vi "PH_Beckhoff_StepMot.ProcCases.vi"(0 "i ref in":refnum<vi>, 1 "selector":string, 2 "Data":T1, 3 "call cluster":T2={"Object"="", "Selector"="", "CallType"=enum."synchronous", "Async Object"="", "Async Selector"="", "Data Descriptor"="", "Data"=[], "Error #"=0, "Expire"=0}, 5 "error in (no error)":errorcluster) -> (14 "i ref out":refnum<vi>, 17 "answer cluster":T2={"Object"="", "Selector"="", "CallType"=enum."synchronous", "Async Object"="", "Async Selector"="", "Data Descriptor"="", "Data"=[], "Error #"=0, "Expire"=0}, 19 "error out":errorcluster)   [LabVIEW 2014, in "PH_Beckhoff_StepMot.lvlib"]
doc: "This method is called by a process from within the default case in the event loop. The methods of a class that are linked to events will be called from THIS method. Add your code here."
uses:
  PH_Beckhoff_StepMot.lvlib
  CS_Core/CSSystem/CoreDefs/CoreDefs.call_type.ctl
  CS_Core/BaseProcess/BaseProcess.descriptor string definition.ctl
  CS_Core/CSSystem/CoreDefs/CoreDefs.rawDataType.ctl
  PH_Beckhoff_StepMot.Axis Cluster.ctl
  instr.lib/Beckhoff/Specials/Step Motor Klemmen/Beckhoff.Step Motor - Motor Configuration.ctl
  instr.lib/Beckhoff/Read and Write Register/Step Motor Klemmen/Beckhoff.Step Motor - Feature Register 1.ctl
  instr.lib/Beckhoff/Read and Write Register/Step Motor Klemmen/Beckhoff.Step Motor - Feature Register 2.ctl
  PH_Basics/PH_PSDBWriter/PH_PSDBWriter.Thread Commands.ctl
  CS_Core/CSSystem/CoreLib/CoreLib.byte array 2 int.vi
  CS_Core/CSSystem/CoreLib/CoreLib.byte array 2 double.vi
  CS_Core/CSSystem/CoreLib/CoreLib.string 2 byte array.vi
  PH_Beckhoff/PH_Beckhoff.lvlib
  CS_Core/CSSystem/CoreLib/CoreLib.lvlib
  CS_Core/BaseProcess/BaseProcess.lvlib
  instr.lib/Beckhoff/Beckhoff - Driver np.lvlib
  PH_Basics/PH_Stepmotor_BaseClass/PH_Stepmotor_BaseClass.lvlib
  PH_Basics/PH_PSDBWriter/PH_PSDBWriter.lvlib
  CS_Core/CAEObj/CAEObj.lvlib
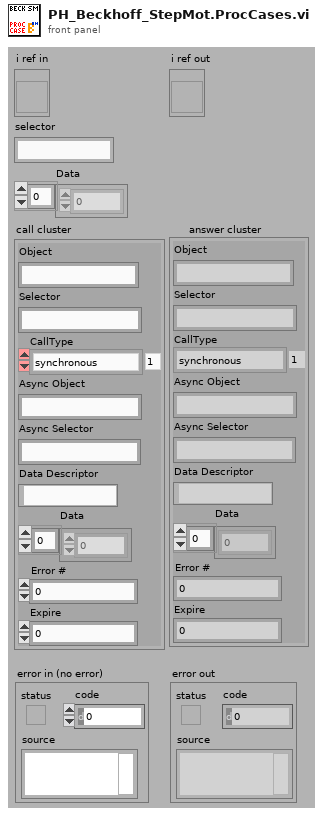
[diagram p1: front panel]
types:
  T1 = typedef "CoreDefs.rawDataType.ctl" = i8[]
  T2 = typedef "CoreDefs.call_type.ctl" = cluster{"Object":string, "Selector":string, "CallType":enum16{"simple", "synchronous", "asynchronous"}, "Async Object":string, "Async Selector":string, "Data Descriptor":T3, "Data":T1, "Error #":i32, "Expire":u32}
  T3 = typedef "BaseProcess.lvlib/BaseProcess.descriptor string definition.ctl" = string
  T4 = typedef "PH_Beckhoff_StepMot.lvlib/PH_Beckhoff_StepMot.Axis Cluster.ctl" = cluster{"Step Motor Configuration":T5, "To set?":bool, "Endswitch inverted?":bool}
  T5 = typedef "Beckhoff - Driver np.lvlib/Beckhoff.Step Motor - Motor Configuration.ctl" = cluster{"Feature Register":T6, "I max A [mA]":dbl, "I max B [mA]":dbl, "v min":u32, "v max":u32, "a max":u32, "I hold [%]":u32, "Steps/qp":u32, "Feature Register 2":T7}
  T6 = typedef "Beckhoff - Driver np.lvlib/Beckhoff.Step Motor - Feature Register 1.ctl" = cluster{"en Auto Start":bool, "en Auto Stop":bool, "dis Wd Timer":bool, "OP Mode 1":bool, "OP Mode 2":bool, "Ramp Type":bool, "inv Pos Feedback":bool, "en User Cur Table":bool, "en Latch Evt Clr Pos":bool, "en Multi Latch Vals":bool, "en Sign Disp*":bool, "Feedback Type*":bool, "en neg Gate Lock*":bool, "en pos Gate Lock*":bool, "dis Enc Fltr*":bool, "en Counter Mode*":bool}
  T7 = typedef "Beckhoff - Driver np.lvlib/Beckhoff.Step Motor - Feature Register 2.ctl" = cluster{"rev Homing Dir":bool, "en Decac Ramp":bool, "Latch Reg Pos":bool, "Show Idle":bool, "dis Ref Input 1":bool, "dis Ref Input 2":bool, "en ext Auto Start":bool, "N/A":bool, "N/A":bool, "N/A":bool, "N/A":bool, "N/A":bool, "en Clr Proc Data":bool, "en Man Ecl Tolerce*":bool, "rev Dig Input 1":bool, "rev Dig Input 2":bool}
  T8 = typedef "PH_Beckhoff.lvlib/PH_Beckhoff.i attribute.ctl" = cluster{"GUI Refs":T9, "operation?":bool, "Default Prdc Interval":i32, "Connection":T10, "AMS Net ID":T11, "Klemmencluster: # of":T12, "Values":T13, "IP":string, "Description":string, "configured?":bool, "Change Manager":cluster{"Detemination wanted?":bool, "Values changed at":cluster{"Sonderklemmen Inputs":i32[], "Analog Inputs":i32[], "Analog Outputs":i32[], "Digital Inputs":i32[], "Digital Outputs":i32[]}}, "Difference to handle an analog input as change":u32}
  T9 = typedef "PH_Beckhoff.lvlib/PH_Beckhoff.GUI Refs.ctl" = cluster{"ADS Error":refnum<vi>, "Values":refnum<vi>, "configured?":refnum<vi>, "Connection":refnum<vi>, "IP":refnum<vi>, "Prdc Int [ms]":refnum<vi>}
  T10 = typedef "PH_Beckhoff.lvlib/PH_Beckhoff.Connectivity.ctl" = cluster{"DLL?":bool, "Port?":bool, "Client?":bool, "Ping?":bool, "unsuccessful Pings":u32}
  T11 = typedef "Beckhoff - Driver np.lvlib/Beckhoff Access.ctl" = cluster{"DLL path":path, "AMS Net ID":cluster{"1st # of IP":u8, "2nd # of IP":u8, "3rd # of IP":u8, "4th # of IP":u8, "In Port":u8, "Out Port":u8}}
  T12 = typedef "Beckhoff - Driver np.lvlib/Klemmendeclarer.ctl" = cluster{"Offset due to Sonderklemms":u32, "analog Inputs":u32, "analog Outputs":u32, "digital Input Bits":u32, "digital Output Bits":u32}
  T13 = typedef "PH_Beckhoff.lvlib/PH_Beckhoff.Values.ctl" = cluster{"Sonderklemmen Inputs":T14, "Analog Inputs":T15, "Analog Outputs":T17, "Digital Inputs":T18, "Digital Outputs":T19}
  T14 = typedef "PH_Beckhoff.lvlib/PH_Beckhoff.Sonderklemmen Inputs.ctl" = cluster{"Total Length":u32, "Name":string, "Value":u64, "Quality":bool, "Service ID":i32, "Offset":u32, "Length":u32}[]
  T15 = typedef "PH_Beckhoff.lvlib/PH_Beckhoff.Analog Inputs.ctl" = cluster{"Name":string, "Value":u32, "Quality":bool, "Service ID":i32, "Sca Type":T16}[]
  T16 = typedef "PH_Beckhoff.lvlib/PH_Beckhoff.Scaling Type.ctl" = enum16{"none", "0 ... 15 Bit -> 0 ... 5", "0 ... 15 Bit -> 0 ... 10", "0 ... 15 Bit -> 0 ... 25", "0 ... 15 Bit -> 4 ... 20", "0 ... 15 Bit -> 0 ... 1", "0 ... 15 Bit -> 0 ... 20000", "0 ... 15 Bit -> 0 ... 24000"}
  T17 = typedef "PH_Beckhoff.lvlib/PH_Beckhoff.Analog Outputs.ctl" = cluster{"Name":string, "Value":u32, "Quality":bool, "Wanted Value":u32, "Service ID":i32, "Sca Type":T16}[]
  T18 = typedef "PH_Beckhoff.lvlib/PH_Beckhoff.Digital Inputs.ctl" = cluster{"Name":string, "Value":bool, "Quality":bool, "Service ID":i32, "inverted?":bool}[]
  T19 = typedef "PH_Beckhoff.lvlib/PH_Beckhoff.Digital Outputs.ctl" = cluster{"Name":string, "Value":bool, "Quality":bool, "Wanted Value":bool, "Service ID":i32, "inverted?":bool}[]
  T20 = cluster{"Boolean array[0]":bool, "Boolean array[1]":bool, "Boolean array[2]":bool, "Boolean array[3]":bool, "Boolean array[4]":bool, "Boolean array[5]":bool, "Boolean array[6]":bool, "Boolean array[7]":bool, "Boolean array[8]":bool, "Boolean array[9]":bool, "Boolean array[10]":bool, "Boolean array[11]":bool, "Boolean array[12]":bool, "Boolean array[13]":bool, "Boolean array[14]":bool, "Boolean array[15]":bool}
  T21 = typedef "PH_PSDBWriter.lvlib/PH_PSDBWriter.PHELIX-Subsystems.ctl" = i32
  T22 = typedef "PH_PSDBWriter.lvlib/PH_PSDBWriter.Thread Commands.ctl" = u16
  T23 = typedef "PH_Stepmotor_BaseClass.lvlib/PH_Stepmotor_BaseClass.i attribute.ctl" = cluster{"Device Error":errorcluster, "Axes PSDB Thread":cluster{"Ref":refnum<vi>, "Q-Ref":refnum<queue>, "Data Status":T24}, "Axes":T25[], "Axes PSDB Infos":cluster{"GUI Name":string, "PSDB Instance ID":i32, "PSDB Status Service ID":i32, "Axis":i32, "Class":string}[], "GUI Refs":T30}
  T24 = typedef "PH_PSDBWriter.lvlib/PH_PSDBWriter.Data Status.ctl" = i16
  T25 = typedef "PH_Stepmotor_BaseClass.lvlib/PH_Stepmotor_BaseClass.Axis Attributes.ctl" = cluster{"Settings":T26, "Endswitch?":bool, "DIM Service IDs":T28, "Activity":T29, "Configured?":bool, "Position":cluster{"Current":i32, "Target":i32}, "Position to set":cluster{"New?":bool, "Wanted":i32}, "Stop?":bool, "Reset?":bool, "Move?":bool, "Nothing connected?":bool}
  T26 = typedef "PH_Stepmotor_BaseClass.lvlib/PH_Stepmotor_BaseClass.Axis Settings.ctl" = cluster{"Sign change":bool, "Width":dbl, "Calibration":dbl, "Unit":string, "Motor Type":T27, "Unit Width":string, "Unit CF":string}
  T27 = typedef "PH_Stepmotor_BaseClass.lvlib/PH_Stepmotor_BaseClass.Motor Type.ctl" = enum16{"Unspecific", "OWIS 49.120.2633", "OWIS 49.060.1033", "OWIS 43.040.2558", "Diamond Motion 2200 series", "OWIS 49.120.266B.MV6", "Calorimeter", "Linear Stage 1", "MICOS VT-80", "MICOS VT-80 S", "Standa Rotstage nt0.95A", "PUF RA 320.200", "PUF RA 800.200", "PUF RA 800.400", "PUF RA 400.50", "1324.nn.800.50", "1324.n9c.800.50", "1324.nn.320.200", "1324.nn.400.200", "1324.nn.800.200", "1324.nn.400.50", "1324.8c9c.800.50", "1324.8c9c.400.200"}
  T28 = typedef "PH_Stepmotor_BaseClass.lvlib/PH_Stepmotor_BaseClass.Axis DIM Service IDs.ctl" = cluster{"Settings":i32, "Information":i32}
  T29 = typedef "PH_Stepmotor_BaseClass.lvlib/PH_Stepmotor_BaseClass.Axis Activity.ctl" = enum16{"No Information", "stopped", "running", "Failure", "Alarm", "stopped at backward ES", "stopped at foreward ES"}
  T30 = typedef "PH_Stepmotor_BaseClass.lvlib/PH_Stepmotor_BaseClass.GUI Refs.ctl" = cluster{"Axes Configuration":refnum<vi>, "Device Error":refnum<vi>, "Axes PSDB Infos":refnum<vi>}
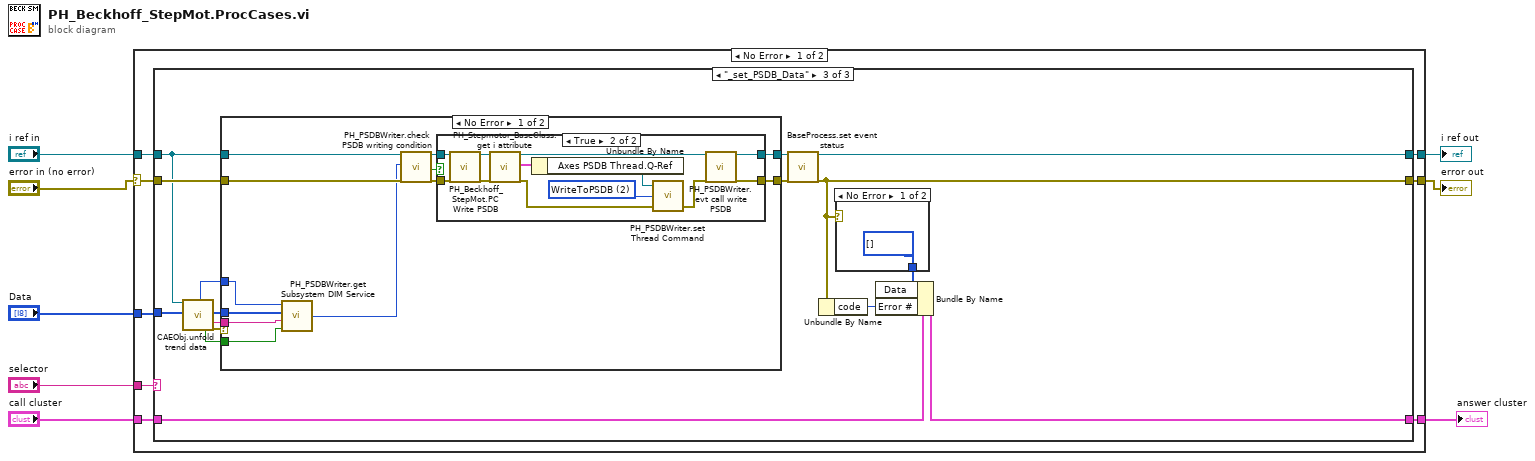
[diagram p0: block diagram]
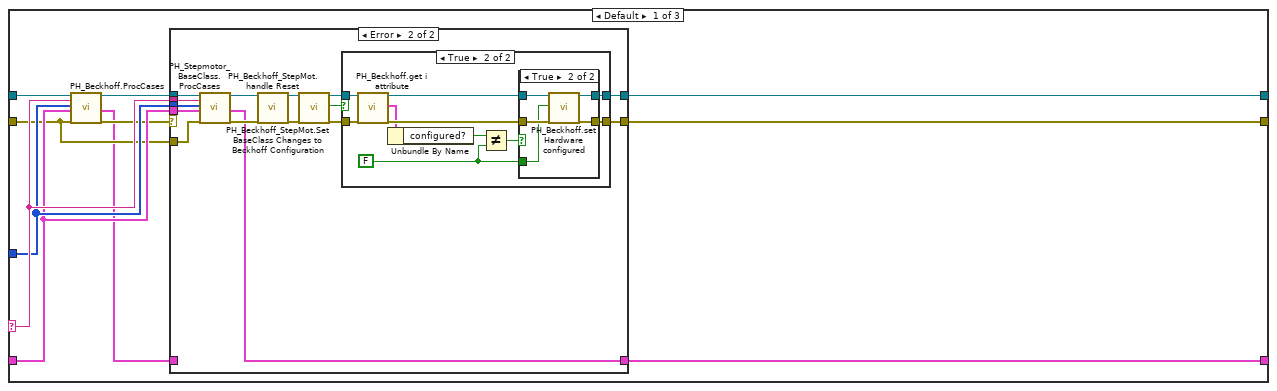
[diagram p2: hidden frame]
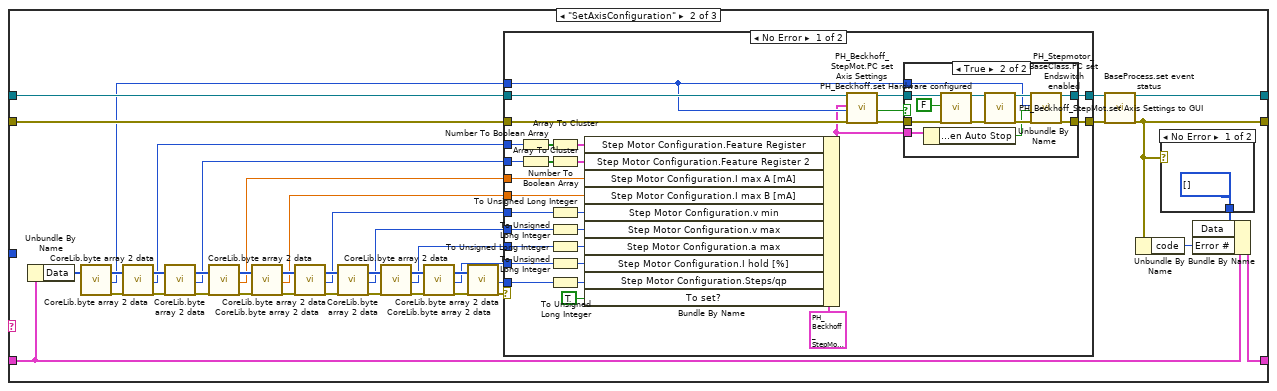
[diagram p6: hidden frame]
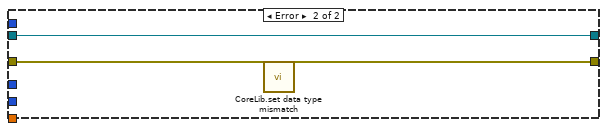
[diagram p8: hidden frame]
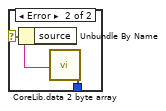
[diagram p9: hidden frame]
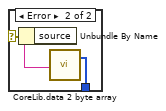
[diagram p12: hidden frame]
diagram:
  n1 = case shown="No Error" "error in (no error)" {
    selector: "error in (no error)" -> [w9 w203]
    tunnel: "selector" -> [w16 _]
    tunnel: [w15 w204] -> w7
    tunnel: "Data" -> [w14 _]
    tunnel: "call cluster" -> [w13 w204]
    tunnel: "i ref in" -> [w12 w205]
    tunnel: [w11 w205] -> w3
    tunnel: [w10 w203] -> w2
    frame No Error {
      n2 = case shown="\"_set_PSDB_Data\"" w16 {
        selector: w16 -> [w23 _ _]
        tunnel: w14 -> [w22 _ w161]
        tunnel: w12 -> [w27 w103 w159]
        tunnel: [w24 w100 w168] -> w11
        tunnel: w13 -> [w21 w95 w165]
        tunnel: [w17 w98 w166] -> w15
        tunnel: w9 -> [w19 w104 w163]
        tunnel: [w26 w99 w167] -> w10
        frame Default {
          n3 = call "PH_Beckhoff.ProcCases.vi"("i ref in"=w27, "selector"=w23, "Data"=w22, "call cluster"=w21, "error in (no error)"=w19) -> ("i ref out"=w25:refnum<vi>, "answer cluster"=w18:T2, "error out"=w20:errorcluster)  [unwired: 12 in]
          n4 = case shown="Error" w20 {
            selector: w20 -> [w29 _]
            tunnel: w19 -> [_ w45]
            tunnel: [w29 w32] -> w26
            tunnel: w25 -> [w30 w43]
            tunnel: [w30 w34] -> w24
            tunnel: w23 -> [_ w42]
            tunnel: w22 -> [_ w41]
            tunnel: w21 -> [_ w40]
            tunnel: [w28 w39] -> w17
            tunnel: w18 -> [w28 _]
            frame No Error {
            }
            frame Error {
              n5 = call "PH_Stepmotor_BaseClass.ProcCases.vi"("i ref in"=w43, "selector"=w42, "Data"=w41, "call cluster"=w40, "error in"=w45) -> ("i ref out"=w36:refnum<vi>, "answer cluster"=w39:T2, "error out"=w44:errorcluster)  [unwired: 12 in]
              n6 = call "PH_Beckhoff_StepMot.handle Reset.vi"("VI in"=w36, "error in (no error)"=w44) -> ("VI out"=w35:refnum<vi>, "error out"=w37:errorcluster)  [unwired: 16 in]
              n7 = call "PH_Beckhoff_StepMot.Set BaseClass Changes to Beckhoff Configuration.vi"("i ref in"=w35, "error in"=w37) -> ("i ref out"=w33:refnum<vi>, "Config changed?"=w31:bool, "error out"=w38:errorcluster)  [unwired: 15 in]
              n8 = case shown="True" w31 {
                tunnel: w38 -> [w46 w57]
                tunnel: [w47 w56] -> w34
                tunnel: w33 -> [w47 w54]
                tunnel: [w46 w55] -> w32
                frame False {
                }
                frame True {
                  w49 = FALSE ("configured?")
                  n9 = call "PH_Beckhoff.get i attribute.vi"("i ref in"=w54, "error in (no error)"=w57) -> ("i ref out"=w53:refnum<vi>, "i attribute"=w51:T8, "error out"=w52:errorcluster)  [unwired: 15 in]
                  n10 = Unbundle By Name(w51) -> ("configured?"=w50:bool)
                  n11 = Not Equal?(x=w50, y=w49) -> (x != y?=w48:bool)
                  n12 = case shown="True" w48 {
                    tunnel: [w59 w64] -> w56
                    tunnel: [w58 w63] -> w55
                    tunnel: w53 -> [w59 w62]
                    tunnel: w52 -> [w58 w61]
                    tunnel: w49 -> [_ w60]
                    frame False {
                    }
                    frame True {
                      n13 = call "PH_Beckhoff.set Hardware configured.vi"("i ref in"=w62, "Hardware configured?"=w60, "error in"=w61) -> ("i ref out"=w64:refnum<vi>, "error out"=w63:errorcluster)  [unwired: 15 in]
                    }
                  }
                }
              }
            }
          }
        }
        frame "SetAxisConfiguration" {
          n14 = Unbundle By Name(w95) -> ("Data"=w68:T1)
          n15 = call-poly "CoreLib.byte array 2 data.vi"("byteArray"=w68) -> ("byteArray out"=w67:T1, "i32"=w65:i32, "error out"=w66:errorcluster)  [unwired: 16 in]
          n16 = call-poly "CoreLib.byte array 2 data.vi"("byteArray"=w67, "error in (no error)"=w66) -> ("byteArray out"=w96:T1, "i32"=w78:i32, "error out"=w97:errorcluster)  [unwired: 15 in]
          n17 = call-poly "CoreLib.byte array 2 data.vi"("byteArray"=w96, "error in (no error)"=w97) -> ("byteArray out"=w82:T1, "i32"=w77:i32, "error out"=w86:errorcluster)  [unwired: 15 in]
          n18 = call-poly "CoreLib.byte array 2 data.vi"("byteArray"=w82, "error in (no error)"=w86) -> ("byteArray out"=w91:T1, "d64"=w76:dbl, "error out"=w92:errorcluster)  [unwired: 15 in]
          n19 = call-poly "CoreLib.byte array 2 data.vi"("byteArray"=w91, "error in (no error)"=w92) -> ("byteArray out"=w81:T1, "d64"=w75:dbl, "error out"=w85:errorcluster)  [unwired: 15 in]
          n20 = call-poly "CoreLib.byte array 2 data.vi"("byteArray"=w81, "error in (no error)"=w85) -> ("byteArray out"=w89:T1, "i32"=w74:i32, "error out"=w90:errorcluster)  [unwired: 15 in]
          n21 = call-poly "CoreLib.byte array 2 data.vi"("byteArray"=w89, "error in (no error)"=w90) -> ("byteArray out"=w80:T1, "i32"=w73:i32, "error out"=w84:errorcluster)  [unwired: 15 in]
          n22 = call-poly "CoreLib.byte array 2 data.vi"("byteArray"=w80, "error in (no error)"=w84) -> ("byteArray out"=w87:T1, "i32"=w72:i32, "error out"=w88:errorcluster)  [unwired: 15 in]
          n23 = call-poly "CoreLib.byte array 2 data.vi"("byteArray"=w87, "error in (no error)"=w88) -> ("byteArray out"=w79:T1, "i32"=w71:i32, "error out"=w83:errorcluster)  [unwired: 15 in]
          n24 = call-poly "CoreLib.byte array 2 data.vi"("byteArray"=w79, "error in (no error)"=w83) -> ("i32"=w70:i32, "error out"=w69:errorcluster)  [unwired: 15 in, 1 out]
          n25 = case shown="No Error" w69 {
            tunnel: w104 -> [w133 w150]
            tunnel: w103 -> [w132 w148]
            tunnel: [w130 w149] -> w94
            tunnel: [w128 w148] -> w93
            tunnel: w78 -> [w121 _]
            tunnel: w77 -> [w120 _]
            tunnel: w76 -> [w119 _]
            tunnel: w75 -> [w118 _]
            tunnel: w74 -> [w110 _]
            tunnel: w73 -> [w117 _]
            tunnel: w72 -> [w116 _]
            tunnel: w71 -> [w115 _]
            tunnel: w70 -> [w114 _]
            tunnel: w65 -> [w106 _]
            frame No Error {
              n26 = Number To Boolean Array(number=w121) -> (Boolean array=w125:bool[])
              n27 = Number To Boolean Array(number=w120) -> (Boolean array=w122:bool[])
              n28 = Array To Cluster(array=w125) -> (cluster=w124:T20)
              n29 = Array To Cluster(array=w122) -> (cluster=w123:T20)
              n30 = To Unsigned Long Integer(number=w110) -> (unsigned 32bit integer=w108:u32)
              n31 = To Unsigned Long Integer(number=w117) -> (unsigned 32bit integer=w107:u32)
              n32 = To Unsigned Long Integer(number=w116) -> (unsigned 32bit integer=w109:u32)
              n33 = To Unsigned Long Integer(number=w115) -> (unsigned 32bit integer=w112:u32)
              n34 = To Unsigned Long Integer(number=w114) -> (unsigned 32bit integer=w113:u32)
              n35 = Bundle By Name(cluster=T4 {"Step Motor Configuration"={"Feature Register"={"en Auto Start"=FALSE, "en Auto Stop"=FALSE, "dis Wd Timer"=FALSE, "OP Mode 1"=FALSE, "OP Mode 2"=FALSE, "Ramp Type"=FALSE, "inv Pos Feedback"=FALSE, "en User Cur Table"=FALSE, "en Latch Evt Clr Pos"=FALSE, "en Multi Latch Vals"=FALSE, "en Sign Disp*"=FALSE, "Feedback Type*"=FALSE, "en neg Gate Lock*"=FALSE, "en pos Gate Lock*"=FALSE, "dis Enc Fltr*"=FALSE, "en Counter Mode*"=FALSE}, "I max A [mA]"=0.0, "I max B [mA]"=0.0, "v min"=0, "v max"=0, "a max"=0, "I hold [%]"=0, "Steps/qp"=0, "Feature Register 2"={"rev Homing Dir"=FALSE, "en Decac Ramp"=FALSE, "Latch Reg Pos"=FALSE, "Show Idle"=FALSE, "dis Ref Input 1"=FALSE, "dis Ref Input 2"=FALSE, "en ext Auto Start"=FALSE, "N/A"=FALSE, "N/A"=FALSE, "N/A"=FALSE, "N/A"=FALSE, "N/A"=FALSE, "en Clr Proc Data"=FALSE, "en Man Ecl Tolerce*"=FALSE, "rev Dig Input 1"=FALSE, "rev Dig Input 2"=FALSE}}, "To set?"=FALSE, "Endswitch inverted?"=FALSE} ("Axis Settings"), "Step Motor Configuration.Feature Register"=w124, "Step Motor Configuration.Feature Register 2"=w123, "Step Motor Configuration.I max A [mA]"=w119, "Step Motor Configuration.I max B [mA]"=w118, "Step Motor Configuration.v min"=w108, "Step Motor Configuration.v max"=w107, "Step Motor Configuration.a max"=w109, "Step Motor Configuration.I hold [%]"=w112, "Step Motor Configuration.Steps/qp"=w113, "To set?"=TRUE) -> (w105:T4)
              n36 = call "PH_Beckhoff_StepMot.PC set Axis Settings.vi"("VI in"=w132, "Axis Settings"=w105, "Axis"=w106, "error in (no error)"=w133) -> ("VI out"=w129:refnum<vi>, "Settings changed?"=w127:bool, "error out"=w131:errorcluster)  [unwired: 13 in]
              n37 = case shown="True" w127 {
                tunnel: w131 -> [w134 w147]
                tunnel: [w134 w141] -> w130
                tunnel: w129 -> [w135 w145]
                tunnel: [w135 w139] -> w128
                tunnel: w106 -> [_ w138]
                tunnel: w105 -> [_ w137]
                frame False {
                }
                frame True {
                  n38 = Unbundle By Name(w137) -> ("Step Motor Configuration.Feature Register.en Auto Stop"=w136:bool)
                  n39 = call "PH_Beckhoff.set Hardware configured.vi"("i ref in"=w145, "Hardware configured?"=FALSE, "error in"=w147) -> ("i ref out"=w144:refnum<vi>, "error out"=w146:errorcluster)  [unwired: 15 in]
                  n40 = call "PH_Beckhoff_StepMot.set Axis Settings to GUI.vi"("VI in"=w144, "error in (no error)"=w146) -> ("VI out"=w140:refnum<vi>, "error out"=w142:errorcluster)  [unwired: 16 in]
                  n41 = call "PH_Stepmotor_BaseClass.PC set Endswitch enabled.vi"("VI in"=w140, "axis"=w138, "Endswitch?"=w136, "error in (no error)"=w142) -> ("VI out"=w139:refnum<vi>, "error out"=w141:errorcluster)  [unwired: 14 in]
                }
              }
            }
            frame Error {
              n42 = call "CoreLib.set data type mismatch.vi"("error in (no error)"=w150) -> ("error out"=w149:errorcluster)  [unwired: 18 in]
            }
          }
          n43 = call "BaseProcess.set event status.vi"("i ref in"=w93, "error in (no error)"=w94) -> ("i ref out"=w100:refnum<vi>, "error out"=w99:errorcluster)  [unwired: 15 in, 1 out]
          n44 = Unbundle By Name(w99) -> ("code"=w101:i32)
          n45 = case shown="No Error" w99 {
            selector: w99 -> [_ w154]
            tunnel: [T1 [] ("byteArray out") w152] -> w102
            frame No Error {
            }
            frame Error {
              n46 = Unbundle By Name(w154) -> ("source"=w153:string)
              n47 = call-poly "CoreLib.data 2 byte array.vi"("string"=w153) -> ("byteArray out"=w152:T1)  [unwired: 18 in]
            }
          }
          n48 = Bundle By Name(cluster=w95, "Data"=w102, "Error #"=w101) -> (w98:T2)
        }
        frame "_set_PSDB_Data" {
          n49 = call "CAEObj.unfold trend data.vi"("i ref in"=w159, "raw trend data"=w161) -> ("quality"=w158:i32, "no link"=w155:bool, "data"=w157:i8[], "typeDescriptor"=w156:string, "error out"=w160:errorcluster)  [unwired: 9 in, 4 out]
          n50 = case shown="No Error" w160 {
            tunnel: w159 -> [w179 w198]
            tunnel: [w178 w198] -> w164
            tunnel: w163 -> [w177 w197]
            tunnel: [w176 w197] -> w162
            tunnel: w158 -> [w173 _]
            tunnel: w157 -> [w175 _]
            tunnel: w156 -> [w174 _]
            tunnel: w155 -> [w172 _]
            frame No Error {
              n51 = call "PH_PSDBWriter.get Subsystem DIM Service.vi"("no link"=w172, "typeDescriptor"=w174, "data"=w175, "quality"=w173) -> ("PHELIX Subsystems"=w171:T21)
              n52 = call "PH_PSDBWriter.check PSDB writing condition.vi"("i ref in"=w179, "wanted Subsystem"=w171, "error IO"=w177) -> ("i ref out"=w181:refnum<vi>, "write PSDB?"=w180:bool, "error out"=w182:errorcluster)  [unwired: 14 in]
              n53 = case shown="True" w180 {
                tunnel: w182 -> [w183 w196]
                tunnel: [w184 w187] -> w178
                tunnel: [w183 w185] -> w176
                tunnel: w181 -> [w184 w195]
                frame False {
                }
                frame True {
                  w191 = T22 2 items=["None", "GetInstanceID", "WriteToPSDB"] ("PSDB Thread Command")
                  n54 = call "PH_Beckhoff_StepMot.PC Write PSDB.vi"("i ref in"=w195, "error IO"=w196) -> ("i ref out"=w189:refnum<vi>, "error out"=w190:errorcluster)  [unwired: 16 in]
                  n55 = call "PH_Stepmotor_BaseClass.get i attribute.vi"("i ref in"=w189, "error in (no error)"=w190) -> ("i ref out"=w188:refnum<vi>, "i attribute"=w193:T23, "error out"=w194:errorcluster)  [unwired: 15 in]
                  n56 = Unbundle By Name(w193) -> ("Axes PSDB Thread.Q-Ref"=w192:refnum<queue>)
                  n57 = call "PH_PSDBWriter.set Thread Command.vi"("error in (no error)"=w194, "PSDB Thread Command"=w191, "Queue in"=w192) -> ("error out"=w186:errorcluster)  [unwired: 2 in]
                  n58 = call "PH_PSDBWriter.evt call write PSDB.vi"("i ref in"=w188, "error in (no error)"=w186) -> ("i ref out"=w187:refnum<vi>, "error out"=w185:errorcluster)  [unwired: 16 in]
                }
              }
            }
            frame Error {
            }
          }
          n59 = call "BaseProcess.set event status.vi"("i ref in"=w164, "error in (no error)"=w162) -> ("i ref out"=w168:refnum<vi>, "error out"=w167:errorcluster)  [unwired: 15 in, 1 out]
          n60 = Unbundle By Name(w167) -> ("code"=w169:i32)
          n61 = case shown="No Error" w167 {
            selector: w167 -> [_ w202]
            tunnel: [T1 [] ("byteArray out") w200] -> w170
            frame No Error {
            }
            frame Error {
              n62 = Unbundle By Name(w202) -> ("source"=w201:string)
              n63 = call-poly "CoreLib.data 2 byte array.vi"("string"=w201) -> ("byteArray out"=w200:T1)  [unwired: 18 in]
            }
          }
          n64 = Bundle By Name(cluster=w165, "Data"=w170, "Error #"=w169) -> (w166:T2)
        }
      }
    }
    frame Error {
    }
  }
  "answer cluster" <- w7
  "i ref out" <- w3
  "error out" <- w2
